vi "Hall Example with Single Point IO.vi"() -> ()   [LabVIEW 2011]
uses:
  <vilib>/Platform/TimedLoop/XDataNode/timing_clust.ctl
  <vilib>/Platform/TimedLoop/XDataNode/nitl_modes.ctl
  <vilib>/Platform/TimedLoop/XDataNode/wakeup.ctl
  <vilib>/rvi/DataTransferAndStorage/Container/Common/niFpgaContainerState.ctl
  <vilib>/rvi/DataTransferAndStorage/Container/Common/niFpgaDataTypeControl.ctl
  <vilib>/rvi/DataTransferAndStorage/Container/Common/niFpgaContainerImplementationControl.ctl
  <vilib>/rvi/DataTransferAndStorage/Container/Common/niFpgaContainerArbitrationOptionsControl.ctl
  <vilib>/rvi/DataTransferAndStorage/Container/Common/niFpgaTransferTypeControl.ctl
  <vilib>/rvi/DataTransferAndStorage/Container/Common/niFpgaContainerInitializationParameters.ctl
  <vilib>/rvi/Memory/Memory_Types/niFpgaMemoryInterfaceConfiguration.ctl
  <vilib>/rvi/FIFO/Fifo_Types/niFpgaFifoControlLogicControl.ctl
  <vilib>/rvi/DataTransferAndStorage/Container/Common/niFpgaContainerMetaDataKey.ctl
  <userlib>/AES/FPGA/FPGA TypeDefs/aes_FullyCustomTeeth ActionEngine Enum.ctl
  <userlib>/_NI VeriStand FPGA Support/NI VeriStand RIO Library/Custom Device Components/Engine Simulation/Engine Simulation Globals.vi
  <userlib>/AES/FPGA/FPGA VIs/AES ECU Event Measurement - All Measurements.vi
  <vilib>/rvi/eio/common/nirviEmuTemplateMethod_errors.vi
  <vilib>/rvi/DataTransferAndStorage/Container/Common/niFpgaContainerGetUniqueNameForEmu.vi
  <vilib>/rvi/DataTransferAndStorage/Container/Common/niFpgaContainerSetEmuInfo.vi
  <vilib>/rvi/eio/common/nirviEmuReportErrorAndStop.vi
  <vilib>/rvi/FIFO/Fifo_Resource/nirvififoEmulationSetSize.vi
  <vilib>/Platform/TimedLoop/XDataNode/XDataNode.xnode
  <vilib>/eio/EIONode/EIONode.xnode
  <vilib>/rvi/LocalResourceManager/LocalResourceManager.xnode
  <vilib>/rvi/DataTransferAndStorage/Container/XNode/niFpgaContainer.xnode
  <vilib>/rvi/FIFO/Fifo_Resource/nirvififoEmulationWrite.vi
  <vilib>/rvi/FIFO/Fifo_Resource/nirvififoEmulationRead.vi
  <vilib>/Platform/TimedLoop/XDataNode/XDNodeRunTimeDep.lvlib
  <vilib>/NI Veristand/FPGA/NI_VS FPGA Support.lvlib
  <userlib>/_NI VeriStand FPGA Support/NI VeriStand FPGA Clock Support/NI_VS FPGA Clock Support.lvlib
  <userlib>/AES/FPGA/AES FPGA.lvlib
panel:
  out "ECUEvent.IC 1.End Angle":u64
  out "ECUEvent.IC 2.End Angle":u64
  out "ECUEvent.IC 3.End Angle":u64
  out "ECUEvent.IC 4.End Angle":u64
  out "ECUEvent.IC 5.End Angle":u64
  out "ECUEvent.IC 6.End Angle":u64
  out "ECUEvent.IC 7.End Angle":u64
  out "ECUEvent.IC 8.End Angle":u64
  out "ECUEvent.IC 1.Time Duration":u32
  out "ECUEvent.IC 1.Start Angle":u64
  out "ECUEvent.IC 1.Angle Duration":u64
  out "ECUEvent.IC 2.Time Duration":u32
  out "ECUEvent.IC 2.Start Angle":u64
  out "ECUEvent.IC 2.Angle Duration":u64
  out "ECUEvent.IC 3.Time Duration":u32
  out "ECUEvent.IC 3.Start Angle":u64
  out "ECUEvent.IC 3.Angle Duration":u64
  out "ECUEvent.IC 4.Time Duration":u32
  out "ECUEvent.IC 4.Start Angle":u64
  out "ECUEvent.IC 4.Angle Duration":u64
  out "ECUEvent.IC 5.Time Duration":u32
  out "ECUEvent.IC 5.Start Angle":u64
  out "ECUEvent.IC 5.Angle Duration":u64
  out "ECUEvent.IC 6.Time Duration":u32
  out "ECUEvent.IC 6.Start Angle":u64
  out "ECUEvent.IC 6.Angle Duration":u64
  out "ECUEvent.IC 7.Time Duration":u32
  out "ECUEvent.IC 7.Start Angle":u64
  out "ECUEvent.IC 7.Angle Duration":u64
  out "ECUEvent.IC 8.Time Duration":u32
  out "ECUEvent.IC 8.Start Angle":u64
  out "ECUEvent.IC 8.Angle Duration":u64
  out "ECUEvent.FI 1.End Angle":u64
  out "ECUEvent.FI 2.End Angle":u64
  out "ECUEvent.FI 3.End Angle":u64
  out "ECUEvent.FI 4.End Angle":u64
  out "ECUEvent.FI 5.End Angle":u64
  out "ECUEvent.FI 6.End Angle":u64
  out "ECUEvent.FI 7.End Angle":u64
  out "ECUEvent.FI 8.End Angle":u64
  out "ECUEvent.FI 1.Time Duration":u32
  out "ECUEvent.FI 1.Start Angle":u64
  out "ECUEvent.FI 1.Angle Duration":u64
  out "ECUEvent.FI 2.Time Duration":u32
  out "ECUEvent.FI 2.Start Angle":u64
  out "ECUEvent.FI 2.Angle Duration":u64
  out "ECUEvent.FI 3.Time Duration":u32
  out "ECUEvent.FI 3.Start Angle":u64
  out "ECUEvent.FI 3.Angle Duration":u64
  out "ECUEvent.FI 4.Time Duration":u32
  out "ECUEvent.FI 4.Start Angle":u64
  out "ECUEvent.FI 4.Angle Duration":u64
  out "ECUEvent.FI 5.Time Duration":u32
  out "ECUEvent.FI 5.Start Angle":u64
  out "ECUEvent.FI 5.Angle Duration":u64
  out "ECUEvent.FI 6.Time Duration":u32
  out "ECUEvent.FI 6.Start Angle":u64
  out "ECUEvent.FI 6.Angle Duration":u64
  out "ECUEvent.FI 7.Time Duration":u32
  out "ECUEvent.FI 7.Start Angle":u64
  out "ECUEvent.FI 7.Angle Duration":u64
  out "ECUEvent.FI 8.Time Duration":u32
  out "ECUEvent.FI 8.Start Angle":u64
  out "ECUEvent.FI 8.Angle Duration":u64
  in  "FullyCustomTeeth.Cams.Cam1.First Rising?":bool
  in  "FullyCustomTeeth.Cams.Num Angles":u8=2
  in  "FullyCustomTeeth.Cams.Cam1.Offset":u64
  in  "FullyCustomTeeth.Cams.Cam2.Offset":u64
  in  "FullyCustomTeeth.Cams.Cam3.Offset":u64
  in  "FullyCustomTeeth.Cams.Cam4.Offset":u64
  in  "FullyCustomTeeth.Cams.Num Profiles":u8=1
  in  "FullyCustomTeeth.Cams.Cam2.First Rising?":bool
  in  "FullyCustomTeeth.Cams.Cam3.First Rising?":bool
  in  "FullyCustomTeeth.Cams.Cam4.First Rising?":bool
  in  "FullyCustomTeeth.Cams.Cam1.CycleAngle":bool=TRUE
  in  "FullyCustomTeeth.Cams.Cam2.CycleAngle":bool=TRUE
  in  "FullyCustomTeeth.Cams.Cam3.CycleAngle":bool=TRUE
  in  "FullyCustomTeeth.Cams.Cam4.CycleAngle":bool=TRUE
  in  "FullyCustomTeeth.Cams.Data":u64
  in  "FullyCustomTeeth.Cams.Toggle":bool
  in  "NTeeth.Crank.TDC Offset":u64
  in  "NTeeth.Crank.Degrees High Pulse":u64
  in  "NTeeth.Crank.Degrees Low Pulse":u64
  in  "NTeeth.Crank.Num Teeth Miss":u8=2 caption="Num. Crank Teeth Missing"
  in  "NTeeth.Crank.Missing Teeth Offset":u64
  in  "NTeeth.Crank.TopDeadCenter High?":bool=TRUE
  in  "NTeeth.Crank.CycleAngle":bool
  in  "APU.Degrees per Tick":u64
  out "APU.Crank Angle":u64
  out "APU.Cycle Angle":u64
  in  "APU.Reset":bool
  in  "APU.Increment Rate":u64
  out "_PWM In Times":u64[](array[numeric])
  in  "_PWM Pulses 0-7":u64[](array[numeric])=[0, 0, 0, 0, 0, 0, 0, 0]
  in  "Generate IRQ":bool
  in  "Use External Timing":bool
  in  "Write to  RTSI":bool
  in  "Loop Rate (usec)":u32
  in  "Start":bool
  in  "_PWM In 7 timeout":u32=40000
  in  "_PWM In 6 timeout":u32=40000
  in  "_PWM In 5 timeout":u32=40000
  in  "_PWM In 4 timeout":u32=40000
  in  "_PWM In 3 timeout":u32=40000
  in  "_PWM In 2 timeout":u32=40000
  in  "_PWM In 1 timeout":u32=40000
  in  "_PWM In 0 timeout":u32=40000
  # "PWM"
  # "Configuration"
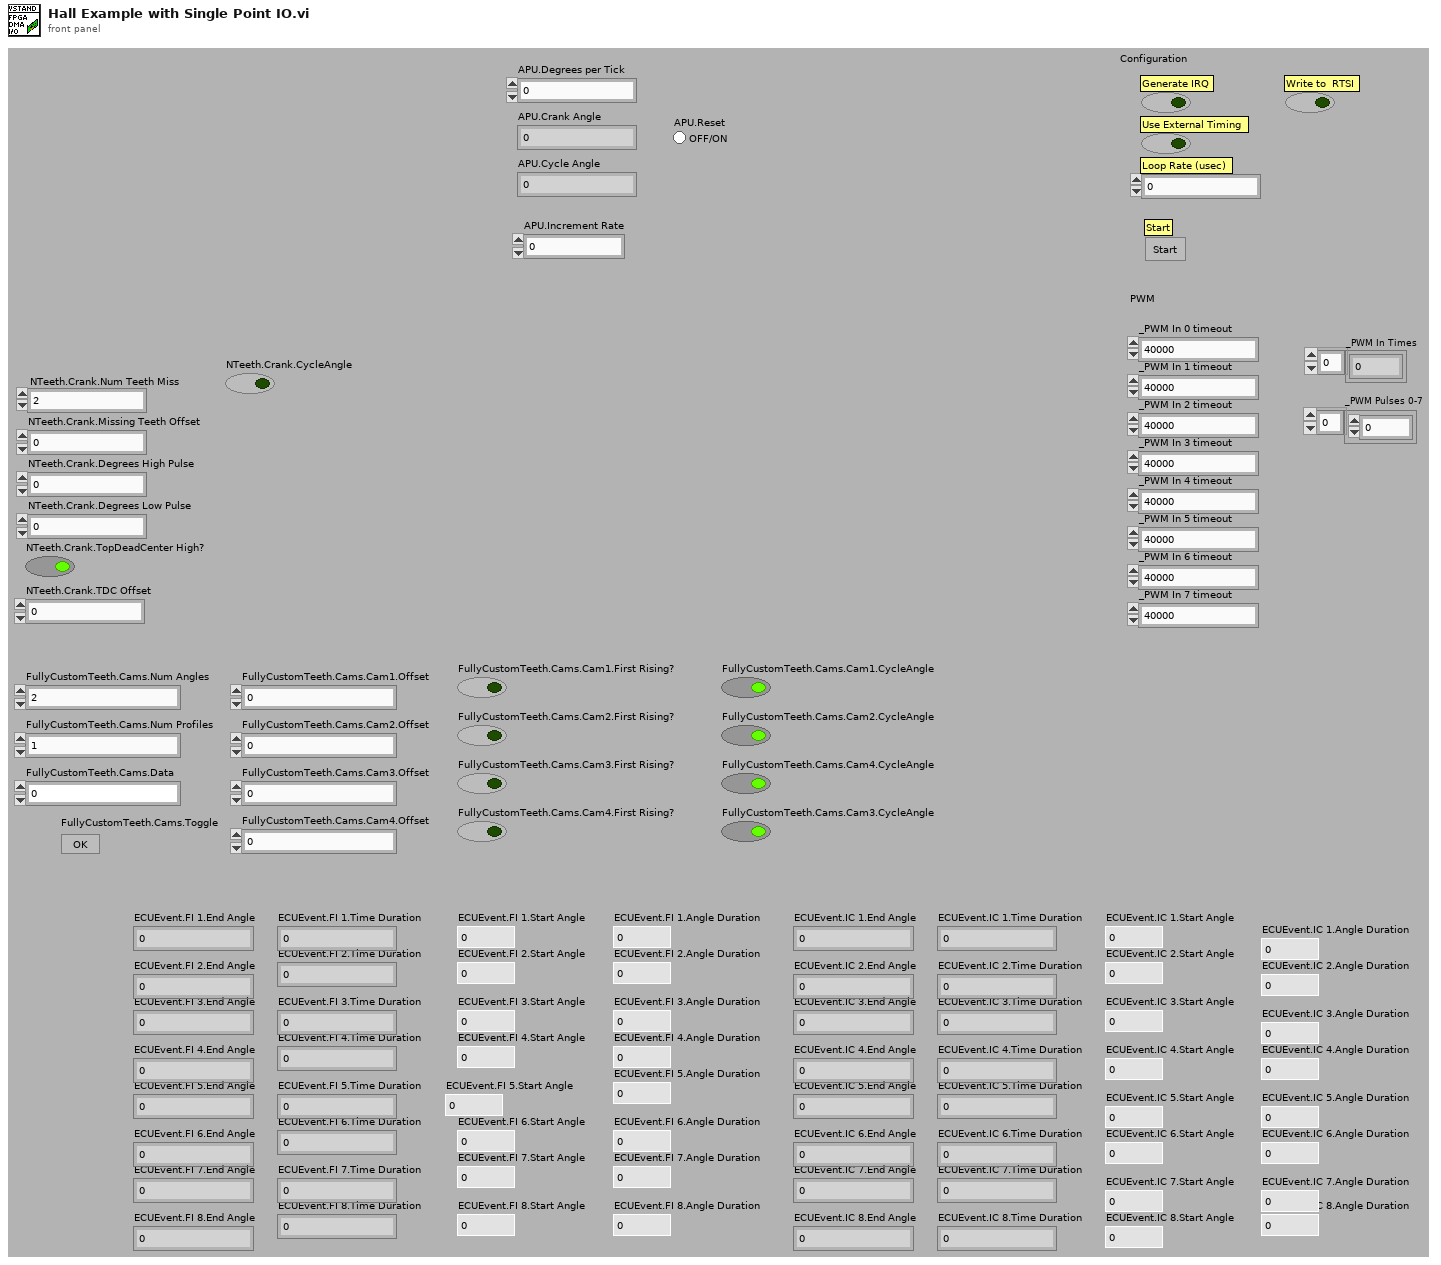
[diagram p1: front panel]
types:
  T1 = typedef "XDNodeRunTimeDep.lvlib/timing_clust.ctl" = cluster{"Expected End [f-1]":u64, "Actual End [f-1]":u64, "Finished Late? [f-1]":bool, "Expected End [i-1]":u64, "Actual End [i-1]":u64, "Finished Late? [i-1]":bool, "Expected Start [i]":u64, "Actual Start [i]":u64, "Expected Start [f]":u64, "Actual Start [f]":u64, "Source Name":string, "Structure Name":string, "Period":i64, "Deadline":i64, "Offset":i64, "Start":i64, "Priority":i32, "Timeout":i32, "Mode":T2, "Wakeup Reason":T3, "Error":errorcluster, "Source Type":string, "Secondary Source Type":string, "Global End Time":u64, "Global Start Time":u64, "Frame Duration":u64, "Iteration Duration":u64, "Assigned CPU":i32, "I/O Scan Engine Mode":u32}
  T2 = typedef "XDNodeRunTimeDep.lvlib/nitl_modes.ctl" = enum32{"No Change", "Process missed periods, maintain original phase", "Discard missed periods, maintain original phase", "Process missed periods, ignore original phase", "Discard missed periods, ignore original phase"}
  T3 = typedef "XDNodeRunTimeDep.lvlib/wakeup.ctl" = enum32{"Normal", "Aborted", "Asynchronous wakeup", "Timing source error", "Timed loop error", "Timeout"}
  T4 = typedef "AES.lvlib/AES FPGA.lvlib/aes_FullyCustomTeeth ActionEngine Enum.ctl" = enum16{"Write Angle", "Update Output"}
  T5 = cluster{"DI0":refnum<k21>, "DI1":refnum<k21>, "DI2":refnum<k21>, "DI3":refnum<k21>, "DI4":refnum<k21>, "DI5":refnum<k21>, "DI6":refnum<k21>, "DI7":refnum<k21>}
  T6 = cluster{"DO0":refnum<k21>, "DO1":refnum<k21>, "DO2":refnum<k21>, "DO3":refnum<k21>, "DO4":refnum<k21>, "DO5":refnum<k21>, "DO6":refnum<k21>, "DO7":refnum<k21>}
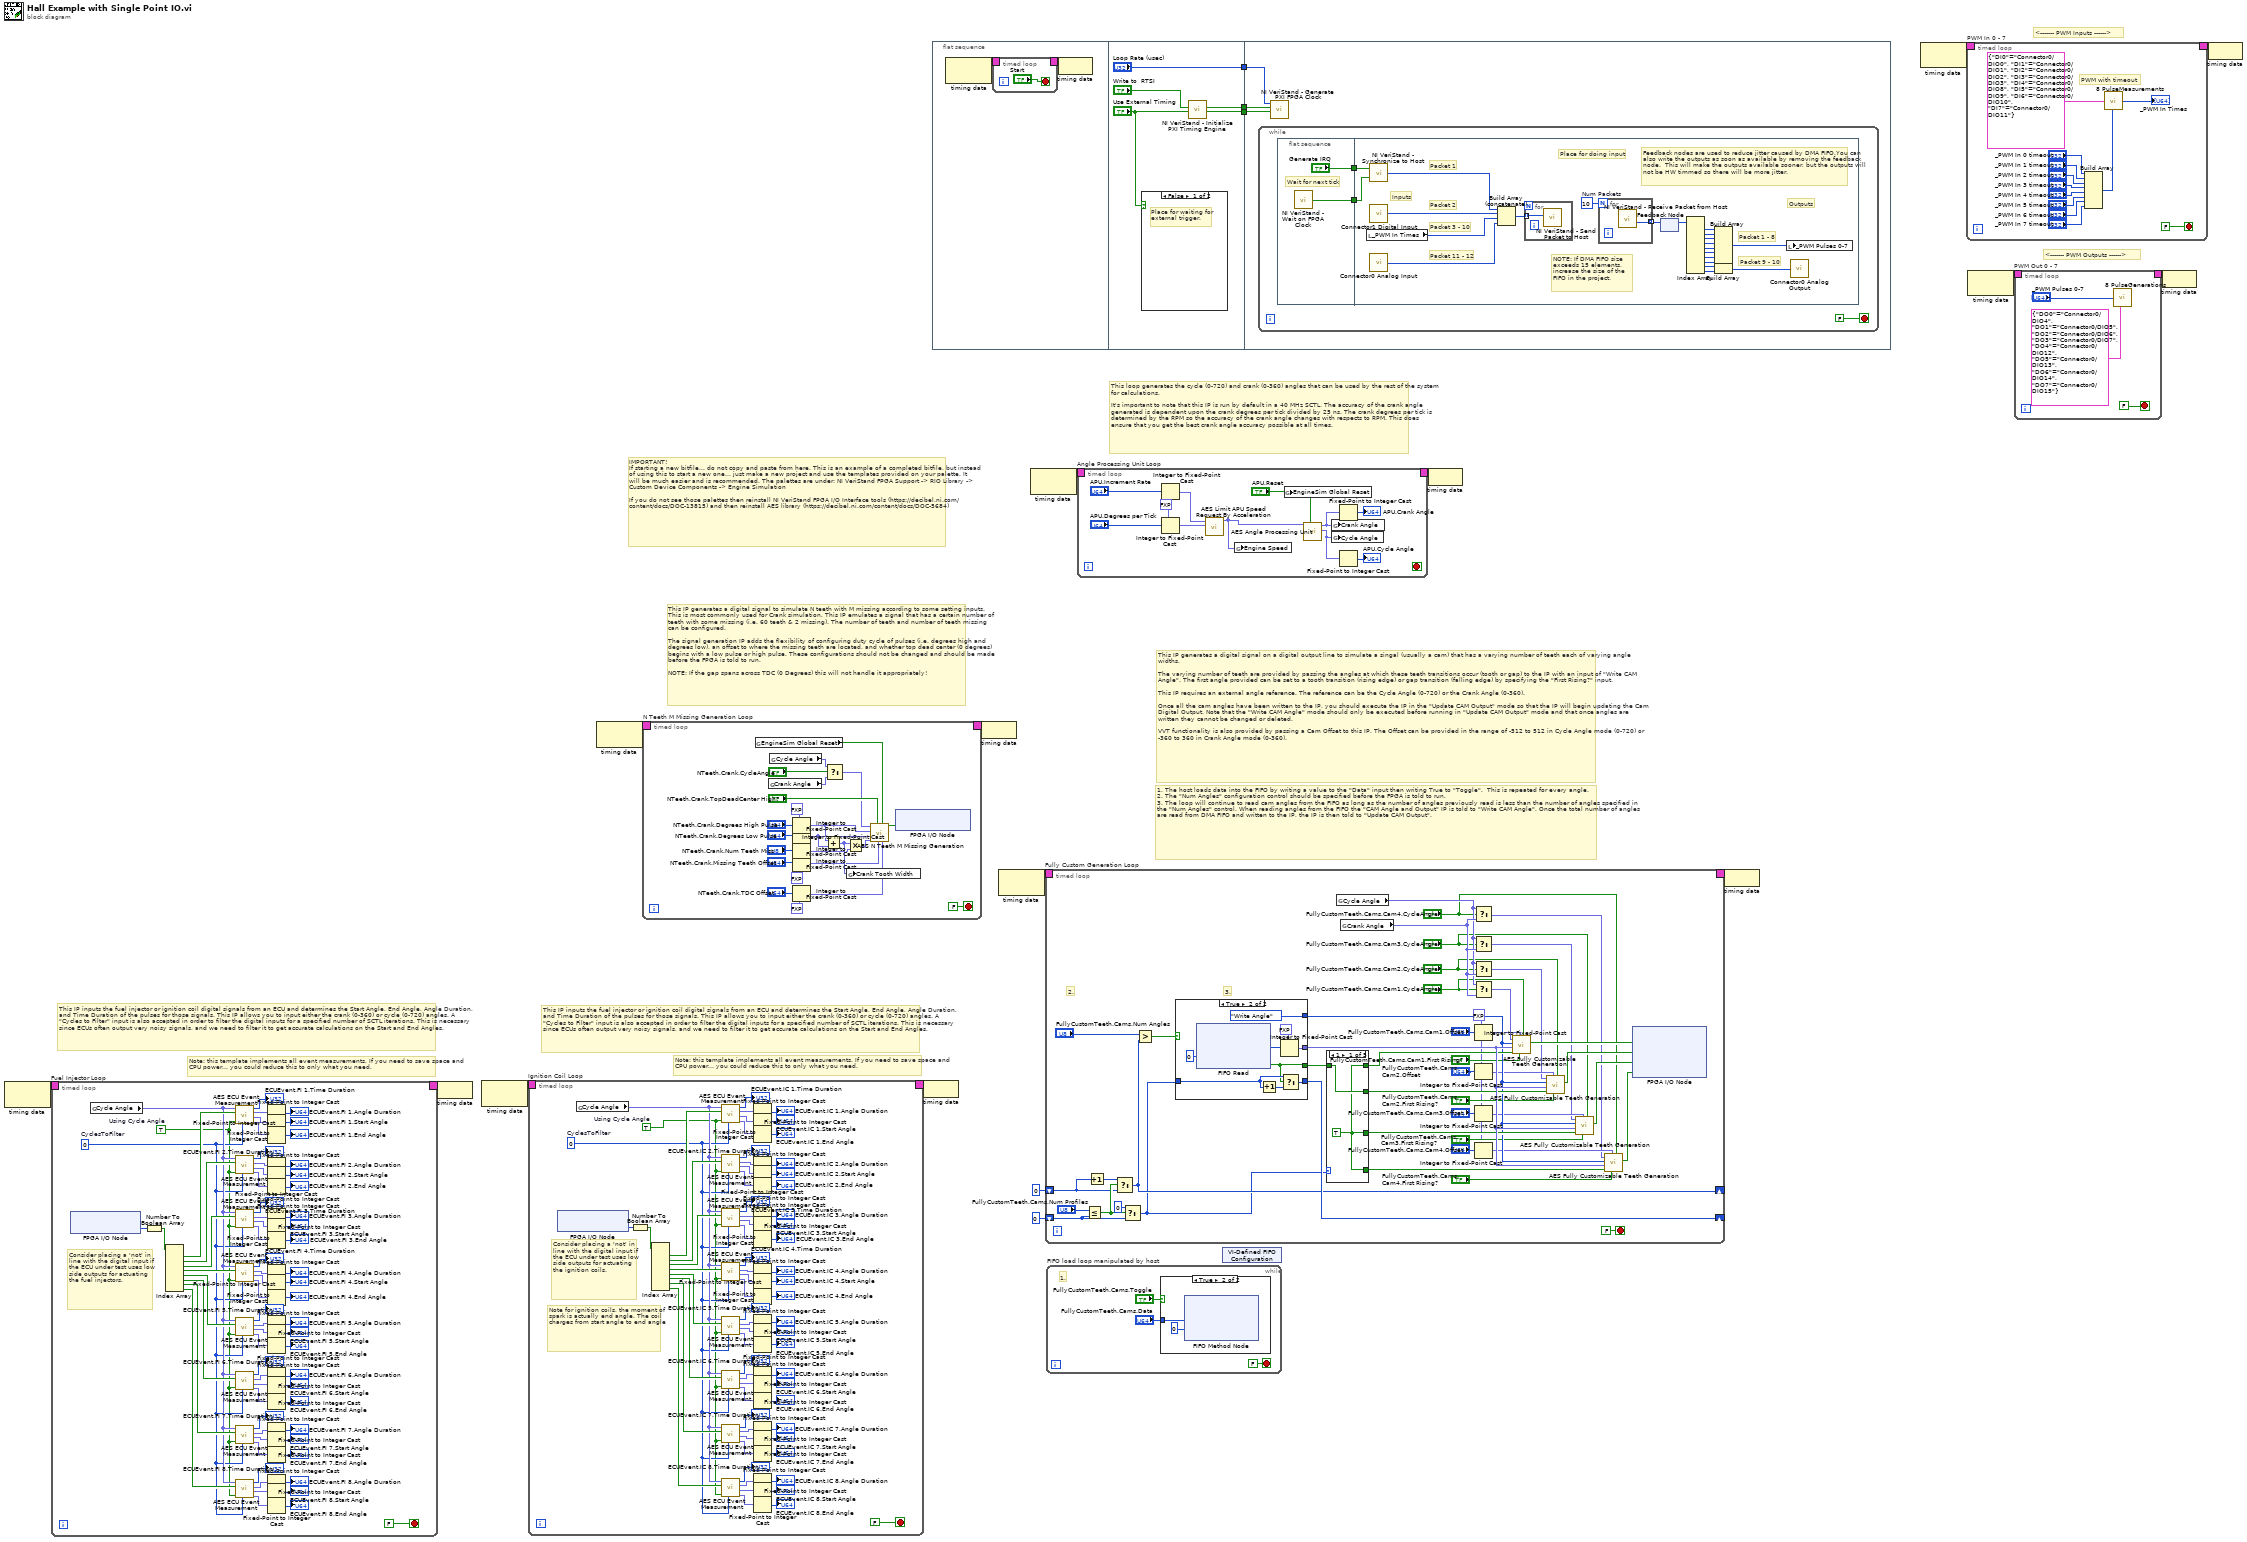
[diagram p0: block diagram]
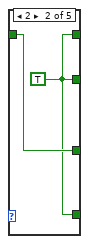
[diagram p3: hidden frame]
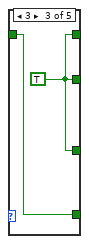
[diagram p4: hidden frame]
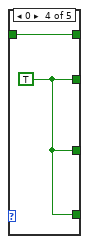
[diagram p5: hidden frame]
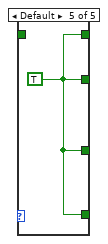
[diagram p6: hidden frame]
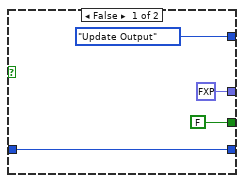
[diagram p7: hidden frame]
diagram:
  # "Note: this template implements all event measurements. If you need to save space and CPU power... you could reduce this to only what you need."
  # "This IP inputs the fuel injector or ignition coil digital signals from an ECU and determines the Start Angle, End Angle, Angle Duration, and Time Duration of the pulses for those signals. This IP allows you to input either the crank (0-360) or cycle (0-720) angles. A \"Cycles to Filter\" input is also accepted in order to filter the digital inputs for a specified number of SCTL iterations. This is necessary since ECUs often output very noisy signals, and we need to filter it to get accurate calculations on the Start and End Angles."
  # "Note: this template implements all event measurements. If you need to save space and CPU power... you could reduce this to only what you need."
  # "This IP inputs the fuel injector or ignition coil digital signals from an ECU and determines the Start Angle, End Angle, Angle Duration, and Time Duration of the pulses for those signals. This IP allows you to input either the crank (0-360) or cycle (0-720) angles. A \"Cycles to Filter\" input is also accepted in order to filter the digital inputs for a specified number of SCTL iterations. This is necessary since ECUs often output very noisy signals, and we need to filter it to get accurate calculations on the Start and End Angles."
  # "1. The host loads data into the FIFO by writing a value to the \"Data\" input then writing True to \"Toggle\".  This is repeated for every angle.\n2. The \"Num Angles\" configuration control should be specified before the FPGA is told to run.\n3. The loop will continue to read cam angles from the FIFO as long as the number of angles previously read is less than the number of angles specified in the \"Num Angles\" control. When reading angles from the FIFO the \"CAM Angle and Output\" IP is told to \"Write CAM Angle\". Once the total number of angles are read from DMA FIFO and written to the IP, the IP is then told to \"Update CAM Output\"."
  # "This IP generates a digital signal on a digital output line to simulate a singal (usually a cam) that has a varying number of teeth each of varying angle widths. \n\nThe varying number of teeth are provided by passing the angles at which these teeth transitions occur (tooth or gap) to the IP with an input of \"Write CAM Angle\". The first angle provided can be set to a tooth transition (rising edge) or gap transition (falling edge) by specifying the \"First Rising?\" input. \n\nThis IP requires an external angle reference. The reference can be the Cycle Angle (0-720) or the Crank Angle (0-360). \n\nOnce all the cam angles have been written to the IP, you should execute the IP in the \"Update CAM Output\" mode so that the IP will begin updating the Cam Digital Output. Note that the \"Write CAM Angle\" mode should only be executed before running in \"Update CAM Output\" mode and that once angles are written they cannot be changed or deleted.\n\nVVT functionality is also provided by passing a Cam Offset to this IP. The Offset can be provided in the range of -512 to 512 in Cycle Angle mode (0-720) or -360 to 360 in Crank Angle mode (0-360)."
  # "This IP generates a digital signal to simulate N teeth with M missing according to some setting inputs. This is most commonly used for Crank simulation. This IP emulates a signal that has a certain number of teeth with some missing (i.e. 60 teeth & 2 missing). The number of teeth and number of teeth missing can be configured. \n\nThe signal generation IP adds the flexibility of configuring duty cycle of pulses (i.e. degrees high and degrees low), an offset to where the missing teeth are located, and whether top dead center (0 degrees) begins with a low pulse or high pulse. These configurations should not be changed and should be made before the FPGA is told to run.\n\nNOTE: If the gap spans across TDC (0 Degrees) this will not handle it appropriately!"
  # "IMPORTANT!\nIf starting a new bitfile... do not copy and paste from here. This is an example of a completed bitfile, but instead of using this to start a new one... just make a new project and use the templates provided on your palette. It will be much easier and is recommended. The palettes are under: NI VeriStand FPGA Support -> RIO Library -> Custom Device Components -> Engine Simulation\n\nIf you do not see those palettes then reinstall NI VeriStand FPGA I/O Interface tools (https://decibel.ni.com/content/docs/DOC-13815) and then reinstall AES library (https://decibel.ni.com/content/docs/DOC-5684)"
  # "This loop generates the cycle (0-720) and crank (0-360) angles that can be used by the rest of the system for calculations. \n\nIt's important to note that this IP is run by default in a 40 MHz SCTL. The accuracy of the crank angle generated is dependent upon the crank degrees per tick divided by 25 ns. The crank degrees per tick is determined by the RPM so the accuracy of the crank angle changes with respects to RPM. This does ensure that you get the best crank angle accuracy possible at all times."
  # "<------- PWM Outputs ------>"
  # "<------- PWM Inputs ------>"
  n1 = node-c288() -> (w4:T1)  [unwired: 1 out]
  n2 = timed-loop "Fuel Injector Loop" {
    timing: w4 -> [_]
    timing-out: [_] -> w3
    stop <- FALSE stop-if-true
    w20 = TRUE  # Using Cycle Angle
    w78 = u16 0  # CyclesToFilter
    # "Consider placing a 'not' in line with the digital input if the ECU under test uses low side outputs for actuating the fuel injectors."
    n3 = xnode "FPGA I/O Node"() -> ("FuelInjector8:1"=w22:u8)  [unwired: 1 in, 1 out]
    n4 = global read "Engine Simulation Globals.vi" "Cycle Angle"() -> (w79:fxp<+,61,10>)
    n5 = Number To Boolean Array(number=w22) -> (Boolean array=w80:bool[])
    n6 = Index Array(array=w80) -> (element #1=w86:bool, element #2=w87:bool, element #3=w88:bool, element #4=w85:bool, element #5=w84:bool, element #6=w83:bool, element #7=w82:bool, element #8=w81:bool)  [unwired: 8 in]
    n7 = call-poly <userlib>:"AES ECU Event Measurement.vi"("Cycles to Filter"=w78, "Using Cycle Angle"=w20, "Digital Input Pulse"=w86, "Crank or Cyle Angle"=w79) -> ("End Angle (degrees)"=w69:fxp<+,61,10>, "Start Angle (degrees)"=w62:fxp<+,61,10>, "Angle Duration (degrees)"=w61:fxp<+/-,62,11>, "Time Duration (clock ticks)"=→"ECUEvent.FI 1.Time Duration":u32)  [unwired: 4 in]
    n8 = call-poly <userlib>:"AES ECU Event Measurement.vi"("Cycles to Filter"=w78, "Using Cycle Angle"=w20, "Digital Input Pulse"=w87, "Crank or Cyle Angle"=w79) -> ("End Angle (degrees)"=w68:fxp<+,61,10>, "Start Angle (degrees)"=w56:fxp<+,61,10>, "Angle Duration (degrees)"=w55:fxp<+/-,62,11>, "Time Duration (clock ticks)"=→"ECUEvent.FI 2.Time Duration":u32)  [unwired: 4 in]
    n9 = call-poly <userlib>:"AES ECU Event Measurement.vi"("Cycles to Filter"=w78, "Using Cycle Angle"=w20, "Digital Input Pulse"=w88, "Crank or Cyle Angle"=w79) -> ("End Angle (degrees)"=w67:fxp<+,61,10>, "Start Angle (degrees)"=w50:fxp<+,61,10>, "Angle Duration (degrees)"=w49:fxp<+/-,62,11>, "Time Duration (clock ticks)"=→"ECUEvent.FI 3.Time Duration":u32)  [unwired: 4 in]
    n10 = call-poly <userlib>:"AES ECU Event Measurement.vi"("Cycles to Filter"=w78, "Using Cycle Angle"=w20, "Digital Input Pulse"=w85, "Crank or Cyle Angle"=w79) -> ("End Angle (degrees)"=w66:fxp<+,61,10>, "Start Angle (degrees)"=w43:fxp<+,61,10>, "Angle Duration (degrees)"=w44:fxp<+/-,62,11>, "Time Duration (clock ticks)"=→"ECUEvent.FI 4.Time Duration":u32)  [unwired: 4 in]
    n11 = call-poly <userlib>:"AES ECU Event Measurement.vi"("Cycles to Filter"=w78, "Using Cycle Angle"=w20, "Digital Input Pulse"=w84, "Crank or Cyle Angle"=w79) -> ("End Angle (degrees)"=w65:fxp<+,61,10>, "Start Angle (degrees)"=w40:fxp<+,61,10>, "Angle Duration (degrees)"=w39:fxp<+/-,62,11>, "Time Duration (clock ticks)"=→"ECUEvent.FI 5.Time Duration":u32)  [unwired: 4 in]
    n12 = call-poly <userlib>:"AES ECU Event Measurement.vi"("Cycles to Filter"=w78, "Using Cycle Angle"=w20, "Digital Input Pulse"=w83, "Crank or Cyle Angle"=w79) -> ("End Angle (degrees)"=w36:fxp<+,61,10>, "Start Angle (degrees)"=w34:fxp<+,61,10>, "Angle Duration (degrees)"=w35:fxp<+/-,62,11>, "Time Duration (clock ticks)"=→"ECUEvent.FI 6.Time Duration":u32)  [unwired: 4 in]
    n13 = call-poly <userlib>:"AES ECU Event Measurement.vi"("Cycles to Filter"=w78, "Using Cycle Angle"=w20, "Digital Input Pulse"=w82, "Crank or Cyle Angle"=w79) -> ("End Angle (degrees)"=w64:fxp<+,61,10>, "Start Angle (degrees)"=w29:fxp<+,61,10>, "Angle Duration (degrees)"=w30:fxp<+/-,62,11>, "Time Duration (clock ticks)"=→"ECUEvent.FI 7.Time Duration":u32)  [unwired: 4 in]
    n14 = call-poly <userlib>:"AES ECU Event Measurement.vi"("Cycles to Filter"=w78, "Using Cycle Angle"=w20, "Digital Input Pulse"=w81, "Crank or Cyle Angle"=w79) -> ("End Angle (degrees)"=w63:fxp<+,61,10>, "Start Angle (degrees)"=w25:fxp<+,61,10>, "Angle Duration (degrees)"=w24:fxp<+/-,62,11>, "Time Duration (clock ticks)"=→"ECUEvent.FI 8.Time Duration":u32)  [unwired: 4 in]
    n15 = Fixed-Point to Integer Cast(1:w61) -> (0:→"ECUEvent.FI 1.Angle Duration":i64)
    n16 = Fixed-Point to Integer Cast(1:w62) -> (0:→"ECUEvent.FI 1.Start Angle":u64)
    n17 = Fixed-Point to Integer Cast(1:w69) -> (0:→"ECUEvent.FI 1.End Angle":u64)
    n18 = Fixed-Point to Integer Cast(1:w55) -> (0:→"ECUEvent.FI 2.Angle Duration":i64)
    n19 = Fixed-Point to Integer Cast(1:w56) -> (0:→"ECUEvent.FI 2.Start Angle":u64)
    n20 = Fixed-Point to Integer Cast(1:w68) -> (0:→"ECUEvent.FI 2.End Angle":u64)
    n21 = Fixed-Point to Integer Cast(1:w49) -> (0:→"ECUEvent.FI 3.Angle Duration":i64)
    n22 = Fixed-Point to Integer Cast(1:w50) -> (0:→"ECUEvent.FI 3.Start Angle":u64)
    n23 = Fixed-Point to Integer Cast(1:w67) -> (0:→"ECUEvent.FI 3.End Angle":u64)
    n24 = Fixed-Point to Integer Cast(1:w44) -> (0:→"ECUEvent.FI 4.Angle Duration":i64)
    n25 = Fixed-Point to Integer Cast(1:w43) -> (0:→"ECUEvent.FI 4.Start Angle":u64)
    n26 = Fixed-Point to Integer Cast(1:w66) -> (0:→"ECUEvent.FI 4.End Angle":u64)
    n27 = Fixed-Point to Integer Cast(1:w39) -> (0:→"ECUEvent.FI 5.Angle Duration":i64)
    n28 = Fixed-Point to Integer Cast(1:w40) -> (0:→"ECUEvent.FI 5.Start Angle":u64)
    n29 = Fixed-Point to Integer Cast(1:w65) -> (0:→"ECUEvent.FI 5.End Angle":u64)
    n30 = Fixed-Point to Integer Cast(1:w35) -> (0:→"ECUEvent.FI 6.Angle Duration":i64)
    n31 = Fixed-Point to Integer Cast(1:w34) -> (0:→"ECUEvent.FI 6.Start Angle":u64)
    n32 = Fixed-Point to Integer Cast(1:w36) -> (0:→"ECUEvent.FI 6.End Angle":u64)
    n33 = Fixed-Point to Integer Cast(1:w30) -> (0:→"ECUEvent.FI 7.Angle Duration":i64)
    n34 = Fixed-Point to Integer Cast(1:w29) -> (0:→"ECUEvent.FI 7.Start Angle":u64)
    n35 = Fixed-Point to Integer Cast(1:w64) -> (0:→"ECUEvent.FI 7.End Angle":u64)
    n36 = Fixed-Point to Integer Cast(1:w24) -> (0:→"ECUEvent.FI 8.Angle Duration":i64)
    n37 = Fixed-Point to Integer Cast(1:w25) -> (0:→"ECUEvent.FI 8.Start Angle":u64)
    n38 = Fixed-Point to Integer Cast(1:w63) -> (0:→"ECUEvent.FI 8.End Angle":u64)
  }
  n39 = node-c288(w3) -> ()
  n40 = node-c288() -> (w2:T1)  [unwired: 1 out]
  n41 = timed-loop "Ignition Coil Loop" {
    timing: w2 -> [_]
    timing-out: [_] -> w1
    stop <- FALSE stop-if-true
    w92 = TRUE  # Using Cycle Angle
    w149 = u16 0  # CyclesToFilter
    # "Note for ignition coils, the moment of spark is actually end angle. The coil charges from start angle to end angle"
    # "Consider placing a 'not' in line with the digital input if the ECU under test uses low side outputs for actuating the ignition coils."
    n42 = xnode "FPGA I/O Node"() -> ("IgnitionCoil8:1"=w151:u8)  [unwired: 1 in, 1 out]
    n43 = global read "Engine Simulation Globals.vi" "Cycle Angle"() -> (w150:fxp<+,61,10>)
    n44 = Number To Boolean Array(number=w151) -> (Boolean array=w152:bool[])
    n45 = Index Array(array=w152) -> (element #1=w158:bool, element #2=w159:bool, element #3=w160:bool, element #4=w157:bool, element #5=w156:bool, element #6=w155:bool, element #7=w154:bool, element #8=w153:bool)  [unwired: 8 in]
    n46 = call-poly <userlib>:"AES ECU Event Measurement.vi"("Cycles to Filter"=w149, "Using Cycle Angle"=w92, "Digital Input Pulse"=w158, "Crank or Cyle Angle"=w150) -> ("End Angle (degrees)"=w140:fxp<+,61,10>, "Start Angle (degrees)"=w133:fxp<+,61,10>, "Angle Duration (degrees)"=w132:fxp<+/-,62,11>, "Time Duration (clock ticks)"=→"ECUEvent.IC 1.Time Duration":u32)  [unwired: 4 in]
    n47 = call-poly <userlib>:"AES ECU Event Measurement.vi"("Cycles to Filter"=w149, "Using Cycle Angle"=w92, "Digital Input Pulse"=w159, "Crank or Cyle Angle"=w150) -> ("End Angle (degrees)"=w139:fxp<+,61,10>, "Start Angle (degrees)"=w127:fxp<+,61,10>, "Angle Duration (degrees)"=w126:fxp<+/-,62,11>, "Time Duration (clock ticks)"=→"ECUEvent.IC 2.Time Duration":u32)  [unwired: 4 in]
    n48 = call-poly <userlib>:"AES ECU Event Measurement.vi"("Cycles to Filter"=w149, "Using Cycle Angle"=w92, "Digital Input Pulse"=w160, "Crank or Cyle Angle"=w150) -> ("End Angle (degrees)"=w138:fxp<+,61,10>, "Start Angle (degrees)"=w121:fxp<+,61,10>, "Angle Duration (degrees)"=w120:fxp<+/-,62,11>, "Time Duration (clock ticks)"=→"ECUEvent.IC 3.Time Duration":u32)  [unwired: 4 in]
    n49 = call-poly <userlib>:"AES ECU Event Measurement.vi"("Cycles to Filter"=w149, "Using Cycle Angle"=w92, "Digital Input Pulse"=w157, "Crank or Cyle Angle"=w150) -> ("End Angle (degrees)"=w137:fxp<+,61,10>, "Start Angle (degrees)"=w114:fxp<+,61,10>, "Angle Duration (degrees)"=w115:fxp<+/-,62,11>, "Time Duration (clock ticks)"=→"ECUEvent.IC 4.Time Duration":u32)  [unwired: 4 in]
    n50 = call-poly <userlib>:"AES ECU Event Measurement.vi"("Cycles to Filter"=w149, "Using Cycle Angle"=w92, "Digital Input Pulse"=w156, "Crank or Cyle Angle"=w150) -> ("End Angle (degrees)"=w136:fxp<+,61,10>, "Start Angle (degrees)"=w111:fxp<+,61,10>, "Angle Duration (degrees)"=w110:fxp<+/-,62,11>, "Time Duration (clock ticks)"=→"ECUEvent.IC 5.Time Duration":u32)  [unwired: 4 in]
    n51 = call-poly <userlib>:"AES ECU Event Measurement.vi"("Cycles to Filter"=w149, "Using Cycle Angle"=w92, "Digital Input Pulse"=w155, "Crank or Cyle Angle"=w150) -> ("End Angle (degrees)"=w107:fxp<+,61,10>, "Start Angle (degrees)"=w105:fxp<+,61,10>, "Angle Duration (degrees)"=w106:fxp<+/-,62,11>, "Time Duration (clock ticks)"=→"ECUEvent.IC 6.Time Duration":u32)  [unwired: 4 in]
    n52 = call-poly <userlib>:"AES ECU Event Measurement.vi"("Cycles to Filter"=w149, "Using Cycle Angle"=w92, "Digital Input Pulse"=w154, "Crank or Cyle Angle"=w150) -> ("End Angle (degrees)"=w135:fxp<+,61,10>, "Start Angle (degrees)"=w100:fxp<+,61,10>, "Angle Duration (degrees)"=w101:fxp<+/-,62,11>, "Time Duration (clock ticks)"=→"ECUEvent.IC 7.Time Duration":u32)  [unwired: 4 in]
    n53 = call-poly <userlib>:"AES ECU Event Measurement.vi"("Cycles to Filter"=w149, "Using Cycle Angle"=w92, "Digital Input Pulse"=w153, "Crank or Cyle Angle"=w150) -> ("End Angle (degrees)"=w134:fxp<+,61,10>, "Start Angle (degrees)"=w96:fxp<+,61,10>, "Angle Duration (degrees)"=w95:fxp<+/-,62,11>, "Time Duration (clock ticks)"=→"ECUEvent.IC 8.Time Duration":u32)  [unwired: 4 in]
    n54 = Fixed-Point to Integer Cast(1:w132) -> (0:→"ECUEvent.IC 1.Angle Duration":i64)
    n55 = Fixed-Point to Integer Cast(1:w133) -> (0:→"ECUEvent.IC 1.Start Angle":u64)
    n56 = Fixed-Point to Integer Cast(1:w140) -> (0:→"ECUEvent.IC 1.End Angle":u64)
    n57 = Fixed-Point to Integer Cast(1:w126) -> (0:→"ECUEvent.IC 2.Angle Duration":i64)
    n58 = Fixed-Point to Integer Cast(1:w127) -> (0:→"ECUEvent.IC 2.Start Angle":u64)
    n59 = Fixed-Point to Integer Cast(1:w139) -> (0:→"ECUEvent.IC 2.End Angle":u64)
    n60 = Fixed-Point to Integer Cast(1:w120) -> (0:→"ECUEvent.IC 3.Angle Duration":i64)
    n61 = Fixed-Point to Integer Cast(1:w121) -> (0:→"ECUEvent.IC 3.Start Angle":u64)
    n62 = Fixed-Point to Integer Cast(1:w138) -> (0:→"ECUEvent.IC 3.End Angle":u64)
    n63 = Fixed-Point to Integer Cast(1:w115) -> (0:→"ECUEvent.IC 4.Angle Duration":i64)
    n64 = Fixed-Point to Integer Cast(1:w114) -> (0:→"ECUEvent.IC 4.Start Angle":u64)
    n65 = Fixed-Point to Integer Cast(1:w137) -> (0:→"ECUEvent.IC 4.End Angle":u64)
    n66 = Fixed-Point to Integer Cast(1:w110) -> (0:→"ECUEvent.IC 5.Angle Duration":i64)
    n67 = Fixed-Point to Integer Cast(1:w111) -> (0:→"ECUEvent.IC 5.Start Angle":u64)
    n68 = Fixed-Point to Integer Cast(1:w136) -> (0:→"ECUEvent.IC 5.End Angle":u64)
    n69 = Fixed-Point to Integer Cast(1:w106) -> (0:→"ECUEvent.IC 6.Angle Duration":i64)
    n70 = Fixed-Point to Integer Cast(1:w105) -> (0:→"ECUEvent.IC 6.Start Angle":u64)
    n71 = Fixed-Point to Integer Cast(1:w107) -> (0:→"ECUEvent.IC 6.End Angle":u64)
    n72 = Fixed-Point to Integer Cast(1:w101) -> (0:→"ECUEvent.IC 7.Angle Duration":i64)
    n73 = Fixed-Point to Integer Cast(1:w100) -> (0:→"ECUEvent.IC 7.Start Angle":u64)
    n74 = Fixed-Point to Integer Cast(1:w135) -> (0:→"ECUEvent.IC 7.End Angle":u64)
    n75 = Fixed-Point to Integer Cast(1:w95) -> (0:→"ECUEvent.IC 8.Angle Duration":i64)
    n76 = Fixed-Point to Integer Cast(1:w96) -> (0:→"ECUEvent.IC 8.Start Angle":u64)
    n77 = Fixed-Point to Integer Cast(1:w134) -> (0:→"ECUEvent.IC 8.End Angle":u64)
  }
  n78 = node-c288() -> (w10:T1)  [unwired: 1 out]
  n79 = timed-loop "N Teeth M Missing Generation Loop" {
    timing: w10 -> [_]
    timing-out: [_] -> w9
    stop <- FALSE stop-if-true
    w181 = fxp<+,60,9> 0.0 ("NTeeth.Crank.Degrees High Pulse")
    n80 = global read "Engine Simulation Globals.vi" "EngineSim Global Reset"() -> (w168:bool)
    n81 = global read "Engine Simulation Globals.vi" "Crank Angle"() -> (w166:fxp<+,60,9>)
    n82 = global read "Engine Simulation Globals.vi" "Cycle Angle"() -> (w165:fxp<+,61,10>)
    n83 = Integer to Fixed-Point Cast(fixed-point type=w181, integer="NTeeth.Crank.Degrees High Pulse") -> (fixed-point=w173:fxp<+,60,9>)
    n84 = Integer to Fixed-Point Cast(fixed-point type=w181, integer="NTeeth.Crank.Degrees Low Pulse") -> (fixed-point=w175:fxp<+,60,9>)
    n85 = Integer to Fixed-Point Cast(integer="NTeeth.Crank.Num Teeth Miss") -> (fixed-point=w180:fxp<+,8,8>)  [unwired: 1 in]
    n86 = Integer to Fixed-Point Cast(fixed-point type=fxp<+,61,10> 0.0 ("NTeeth.Crank.Missing Teeth Offset"), integer="NTeeth.Crank.Missing Teeth Offset") -> (fixed-point=w176:fxp<+,61,10>)
    n87 = Integer to Fixed-Point Cast(fixed-point type=fxp<+/-,61,10> 0.0 ("NTeeth.TDC Offset"), integer="NTeeth.Crank.TDC Offset") -> (fixed-point=w169:fxp<+/-,61,10>)
    n88 = Add(x=w173, y=w175) -> (x+y=w184:fxp<+,61,10>)
    n89 = Select(t=w165, s="NTeeth.Crank.CycleAngle", f=w166) -> (s? t:f=w164:fxp<+,61,10>)
    n90 = Multiply(x=w184, y=w180) -> (x*y=w174:fxp<+,61,10>)
    n91 = global write "Engine Simulation Globals.vi" "Crank Tooth Width"(w184) -> ()
    n92 = call <userlib>:"AES N Teeth M Missing Generation.vi"("NTeeth.TDC Offset"=w169, "NTeeth.Reset"=w168, "NTeeth.Missing Teeth Offset"=w176, "NTeeth.TopDeadCenter High?"="NTeeth.Crank.TopDeadCenter High?", "NTeeth.Missing Teeth Gap"=w174, "NTeeth.Degrees Low Pulse"=w175, "NTeeth.Degrees High Pulse"=w173, "Crank or Cyle Angle"=w164) -> ("NTeeth.Digital Output"=w185:bool)  [unwired: 3 in]
    n93 = xnode "FPGA I/O Node"("CrankDigitalOut"=w185) -> ()  [unwired: 1 in, 1 out]
  }
  n94 = node-c288(w1) -> ()
  n95 = flat-sequence {
    tunnel: [w197] -> w19
    tunnel: ["Loop Rate (usec)"] -> w18
    tunnel: [w196] -> w13
    tunnel: w19 -> [w203]
    tunnel: w18 -> [w202]
    tunnel: w13 -> [w201]
    frame #0 {
      n96 = node-c288() -> (w190:T1)  [unwired: 1 out]
      n97 = timed-loop {
        timing: w190 -> [_]
        timing-out: [_] -> w189
        stop <- "Start" stop-if-true
      }
      n98 = node-c288(w189) -> ()
    }
    frame #1 {
      n99 = case shown="False" "Use External Timing" {
        frame False {
          # "Place for waiting for external trigger."
        }
        frame True {
          # "Do not wait on trigger when externally timed."
        }
      }
      n100 = call <userlib>:"NI VeriStand - Initialize PXI Timing Engine.vi"("Use External Timing In"="Use External Timing", "Write to  RTSI In"="Write to  RTSI") -> ("Use External Timing Out"=w197:bool, "Write to  RTSI Out"=w196:bool)  [unwired: 8 in]
    }
    frame #2 {
      n101 = while {
        stop <- FALSE stop-if-true
        n102 = flat-sequence {
          tunnel: ["Generate IRQ"] -> w205
          tunnel: [w207] -> w204
          tunnel: w205 -> [w230]
          tunnel: w204 -> [w229]
          frame #0 {
            # "Wait for next tick"
            n103 = call <userlib>:"NI VeriStand - Wait on FPGA Clock.vi"() -> ("Clock Ticked"=w207:bool)
          }
          frame #1 {
            w228 = 10  # Num Packets
            # "Packet 1"
            # "Packet 11 - 12"
            # "Inputs"
            # "Outputs"
            # "Packet 3 - 10"
            # "Packet 2"
            # "Packet 9 - 10"
            # "Packet 1 - 8"
            # "NOTE: If DMA FIFO size exceeds 15 elements, increase the size of the FIFO in the project."
            # "Feedback nodes are used to reduce jitter caused by DMA FIFO.You can also write the outputs as soon as available by removing the feedback node.  This will make the outputs available sooner, but the outputs will not be HW timmed so there will be more jitter."
            # "Place for doing input"
            n104 = local read "_PWM In Times"() -> (w218:u64[])
            n105 = call <userlib>:"NI VeriStand - Synchronize to Host.vi"("Clock Ticked"=w229, "Generate IRQ"=w230) -> ("Is Late?"=w219:u64)
            n106 = call <userlib>:"Connector1 Digital Input.vi"() -> ("Packet"=w209:u64)
            n107 = call <userlib>:"Connector0 Analog Input.vi"() -> ("Packets"=w216:u64[])
            n108 = Build Array (concatenate)(w219, w209, w218, w216) -> (w217:u64[])
            n109 = for {
              tunnel: w217 -> [w231] mode=indexing
              n110 = call <vilib>:"NI VeriStand - Send Packet to Host.vi"("Element"=w231) -> ()  [unwired: 2 in, 9 out]
            }
            n111 = for {
              N: w228 -> [_]
              tunnel: [w232] -> w210 mode=indexing
              n112 = call <vilib>:"NI VeriStand - Receive Packet from Host.vi"() -> ("Element"=w232:u64)  [unwired: 2 in, 9 out]
            }
            n113 = feedback-in #1(w210) -> ()
            n114 = feedback #1() -> (w211:u64[])  [unwired: 1 in]
            n115 = Index Array(array=w211) -> (element #1=w227:u64, element #2=w226:u64, element #3=w225:u64, element #4=w224:u64, element #5=w223:u64, element #6=w222:u64, element #7=w221:u64, element #8=w220:u64, element #9=w215:u64, element #10=w214:u64)  [unwired: 10 in]
            n116 = Build Array(w227, w226, w225, w224, w223, w222, w221, w220) -> (w213:u64[])
            n117 = Build Array(w215, w214) -> (w212:u64[])
            n118 = local write "_PWM Pulses 0-7"(w213) -> ()
            n119 = call <userlib>:"Connector0 Analog Output.vi"("Packets"=w212) -> ()
          }
        }
      }
      n120 = call <userlib>:"NI VeriStand - Generate PXI FPGA Clock.vi"("Use External Timing"=w203, "Write to  RTSI"=w201, "Loop Rate (usec)"=w202) -> ()  [unwired: 9 in]
    }
  }
  n121 = node-c288(w9) -> ()
  n122 = node-c288() -> (w8:T1)  [unwired: 1 out]
  n123 = node-c288() -> (w12:T1)  [unwired: 1 in]
  n124 = timed-loop "Fully Custom Generation Loop" {
    timing: w8 -> [_]
    timing-out: [_] -> w7
    shift-right: [w276] -> _
    shift-left: u8 0 -> [w269]
    shift-right: [w268] -> _
    shift-left: u8 0 ("CAM.Num Angles") -> [w270]
    stop <- FALSE stop-if-true
    w243 = fxp<+/-,61,10> 0.0 ("FullyCustomTeeth.Cams.Cam1.Offset")
    # "3."
    # "2."
    n125 = Less Or Equal?(x="FullyCustomTeeth.Cams.Num Profiles", y=w269) -> (x <= y?=w273:bool)
    n126 = Increment(x=w270) -> (x+1=w272:u8)
    n127 = Select(t=w272, s=w273, f=w270) -> (s? t:f=w268:u8)
    n128 = Select(t=u8 0, s=w273, f=w269) -> (s? t:f=w266:u8)
    n129 = Greater?(x="FullyCustomTeeth.Cams.Num Angles", y=w268) -> (0:w277:bool)
    n130 = case shown="True" w277 {
      tunnel: w266 -> [w291 w298]
      tunnel: [w291 w297] -> w276
      tunnel: [FALSE ("Timed Out?") w296] -> w265
      tunnel: [aes_FullyCustomTeeth_ActionEngine_Enum."Update Output" ("FullyCustomTeeth.Action") aes_FullyCustomTeeth_ActionEngine_Enum."Write Angle" ("FullyCustomTeeth.Action")] -> w256
      tunnel: [fxp<+,61,10> 0.0 ("Element") w293] -> w267
      frame False {
      }
      frame True {
        n131 = xnode ("FIFO Read")("Timeout"=0) -> ("Element"=w295:u64, "Timed Out?"=w296:bool)  [unwired: 1 in, 1 out]
        n132 = Increment(x=w298) -> (x+1=w299:u8)
        n133 = Integer to Fixed-Point Cast(fixed-point type=fxp<+,61,10> 0.0 ("Element"), integer=w295) -> (fixed-point=w293:fxp<+,61,10>)
        n134 = Select(t=w298, s=w296, f=w299) -> (s? t:f=w297:u8)
      }
    }
    n135 = case shown="1" w266 {
      tunnel: w265 -> [w280 w282 w283 w286 _]
      tunnel: [w279 w281 w284 w286 w287] -> w264
      tunnel: [w279 w282 w284 w285 w287] -> w262
      tunnel: [w280 w281 w284 w285 w287] -> w263
      tunnel: [w279 w281 w283 w285 w287] -> w261
      frame 1 {
        w279 = TRUE ("Timed Out?")
      }
      frame 2 {
        w281 = TRUE ("Timed Out?")
      }
      frame 3 {
        w284 = TRUE ("Timed Out?")
      }
      frame 0 {
        w285 = TRUE ("Timed Out?")
      }
      frame Default {
        w287 = TRUE ("Timed Out?")
      }
    }
    n136 = global read "Engine Simulation Globals.vi" "Cycle Angle"() -> (w241:fxp<+,61,10>)
    n137 = global read "Engine Simulation Globals.vi" "Crank Angle"() -> (w242:fxp<+,60,9>)
    n138 = Integer to Fixed-Point Cast(fixed-point type=w243, integer="FullyCustomTeeth.Cams.Cam1.Offset") -> (fixed-point=w250:fxp<+/-,61,10>)
    n139 = Integer to Fixed-Point Cast(fixed-point type=w243, integer="FullyCustomTeeth.Cams.Cam2.Offset") -> (fixed-point=w249:fxp<+/-,61,10>)
    n140 = Integer to Fixed-Point Cast(fixed-point type=w243, integer="FullyCustomTeeth.Cams.Cam3.Offset") -> (fixed-point=w246:fxp<+/-,61,10>)
    n141 = Integer to Fixed-Point Cast(fixed-point type=w243, integer="FullyCustomTeeth.Cams.Cam4.Offset") -> (fixed-point=w244:fxp<+/-,61,10>)
    n142 = Select(t=w241, s="FullyCustomTeeth.Cams.Cam4.CycleAngle", f=w242) -> (s? t:f=w233:fxp<+,61,10>)
    n143 = Select(t=w241, s="FullyCustomTeeth.Cams.Cam3.CycleAngle", f=w242) -> (s? t:f=w236:fxp<+,61,10>)
    n144 = Select(t=w241, s="FullyCustomTeeth.Cams.Cam2.CycleAngle", f=w242) -> (s? t:f=w238:fxp<+,61,10>)
    n145 = Select(t=w241, s="FullyCustomTeeth.Cams.Cam1.CycleAngle", f=w242) -> (s? t:f=w239:fxp<+,61,10>)
    n146 = call <userlib>:"AES Fully Customizable Teeth Generation.vi"("Using Cycle Angle"="FullyCustomTeeth.Cams.Cam1.CycleAngle", "FullyCustomTeeth.FirstElement RisingEdge?"="FullyCustomTeeth.Cams.Cam1.First Rising?", "FullyCustomTeeth.Offset"=w250, "Write Timeout?"=w264, "FullyCustomTeeth.Next Angle"=w267, "FullyCustomTeeth.Action"=w256, "Crank or Cyle Angle"=w239) -> ("FullyCustomTeeth.Digital Output"=w257:bool)  [unwired: 4 in]
    n147 = call <userlib>:"AES Fully Customizable Teeth Generation.vi"("Using Cycle Angle"="FullyCustomTeeth.Cams.Cam2.CycleAngle", "FullyCustomTeeth.FirstElement RisingEdge?"="FullyCustomTeeth.Cams.Cam2.First Rising?", "FullyCustomTeeth.Offset"=w249, "Write Timeout?"=w263, "FullyCustomTeeth.Next Angle"=w267, "FullyCustomTeeth.Action"=w256, "Crank or Cyle Angle"=w238) -> ("FullyCustomTeeth.Digital Output"=w258:bool)  [unwired: 4 in]
    n148 = call <userlib>:"AES Fully Customizable Teeth Generation.vi"("Using Cycle Angle"="FullyCustomTeeth.Cams.Cam3.CycleAngle", "FullyCustomTeeth.FirstElement RisingEdge?"="FullyCustomTeeth.Cams.Cam3.First Rising?", "FullyCustomTeeth.Offset"=w246, "Write Timeout?"=w262, "FullyCustomTeeth.Next Angle"=w267, "FullyCustomTeeth.Action"=w256, "Crank or Cyle Angle"=w236) -> ("FullyCustomTeeth.Digital Output"=w259:bool)  [unwired: 4 in]
    n149 = call <userlib>:"AES Fully Customizable Teeth Generation.vi"("Using Cycle Angle"="FullyCustomTeeth.Cams.Cam4.CycleAngle", "FullyCustomTeeth.FirstElement RisingEdge?"="FullyCustomTeeth.Cams.Cam4.First Rising?", "FullyCustomTeeth.Offset"=w244, "Write Timeout?"=w261, "FullyCustomTeeth.Next Angle"=w267, "FullyCustomTeeth.Action"=w256, "Crank or Cyle Angle"=w233) -> ("FullyCustomTeeth.Digital Output"=w260:bool)  [unwired: 4 in]
    n150 = xnode "FPGA I/O Node"("Cam1DigitalOut"=w257, "Cam2DigitalOut"=w258, "Cam3DigitalOut"=w259, "Cam4DigitalOut"=w260) -> ()  [unwired: 4 in, 4 out]
  }
  n151 = while "FIFO load loop manipulated by host" {
    stop <- FALSE stop-if-true
    # "1."
    n152 = case shown="True" "FullyCustomTeeth.Cams.Toggle" {
      tunnel: "FullyCustomTeeth.Cams.Data" -> [_ w307]
      frame False {
      }
      frame True {
        n153 = xnode ("FIFO Method Node")("Element"=w307, "Timeout"=0) -> ()  [unwired: 1 in, 2 out]
      }
    }
  }
  n154 = timed-loop "Angle Processing Unit Loop" {
    timing: w12 -> [_]
    timing-out: [_] -> w11
    stop <- _ stop-if-true
    w310 = fxp<+/-,47,-4> 0.0 ("Crank.Degrees per Tick")
    n155 = Integer to Fixed-Point Cast(fixed-point type=w310, integer="APU.Increment Rate") -> (fixed-point=w309:fxp<+/-,47,-4>)
    n156 = Integer to Fixed-Point Cast(fixed-point type=w310, integer="APU.Degrees per Tick") -> (fixed-point=w312:fxp<+/-,47,-4>)
    n157 = call <userlib>:"AES Limit APU Speed Request By Acceleration.vi"("APU.Degrees per Tick in"=w312, "APU.Increment Rate"=w309) -> ("APU.Degrees per Tick out"=w308:fxp<+/-,47,-4>)  [unwired: 9 in]
    n158 = global write "Engine Simulation Globals.vi" "Engine Speed"(w308) -> ()
    n159 = global write "Engine Simulation Globals.vi" "EngineSim Global Reset"("APU.Reset") -> ()
    n160 = call <userlib>:"AES Angle Processing Unit.vi"("APU.Reset"="APU.Reset", "APU.Degrees per Tick"=w308) -> ("APU.Cycle Angle"=w314:fxp<+,61,10>, "APU.Crank Angle"=w318:fxp<+,60,9>)  [unwired: 8 in]
    n161 = global write "Engine Simulation Globals.vi" "Crank Angle"(w318) -> ()
    n162 = global write "Engine Simulation Globals.vi" "Cycle Angle"(w314) -> ()
    n163 = Fixed-Point to Integer Cast(1:w318) -> (0:→"APU.Crank Angle":u64)
    n164 = Fixed-Point to Integer Cast(1:w314) -> (0:→"APU.Cycle Angle":u64)
  }
  n165 = xnode "VI-Defined FIFO Configuration"() -> ()  [unwired: 1 out]
  n166 = node-c288(w11) -> ()
  n167 = node-c288(w7) -> ()
  n168 = node-c288() -> (w15:T1)  [unwired: 1 out]
  n169 = timed-loop "PWM In 0 - 7" {
    timing: w15 -> [_]
    timing-out: [_] -> w14
    stop <- FALSE stop-if-true
    # "PWM with timeout"
    n170 = Build Array("_PWM In 0 timeout", "_PWM In 1 timeout", "_PWM In 2 timeout", "_PWM In 3 timeout", "_PWM In 4 timeout", "_PWM In 5 timeout", "_PWM In 6 timeout", "_PWM In 7 timeout") -> (w331:u32[])
    n171 = call <userlib>:"8 PulseMeasurements.vi"("8 PulseMeas Chs"=T5 {"DI0"="Connector0/DIO0", "DI1"="Connector0/DIO1", "DI2"="Connector0/DIO2", "DI3"="Connector0/DIO3", "DI4"="Connector0/DIO8", "DI5"="Connector0/DIO9", "DI6"="Connector0/DIO10", "DI7"="Connector0/DIO11"} ("8 PWM In Chs"), "PulseMeas Timeouts"=w331) -> ("PulseMeas Packets"=→"_PWM In Times":u64[])  [unwired: 7 in]
  }
  n172 = node-c288() -> (w17:T1)  [unwired: 1 out]
  n173 = timed-loop "PWM Out 0 - 7" {
    timing: w17 -> [_]
    timing-out: [_] -> w16
    stop <- FALSE stop-if-true
    n174 = call <userlib>:"8 PulseGenerations.vi"("PulseGen Packets"="_PWM Pulses 0-7", "8 PulseGen Chs"=T6 {"DO0"="Connector0/DIO4", "DO1"="Connector0/DIO5", "DO2"="Connector0/DIO6", "DO3"="Connector0/DIO7", "DO4"="Connector0/DIO12", "DO5"="Connector0/DIO13", "DO6"="Connector0/DIO14", "DO7"="Connector0/DIO15"} ("8 PWM Out Chs")) -> ()  [unwired: 8 in]
  }
  n175 = node-c288(w16) -> ()
  n176 = node-c288(w14) -> ()
